vi "GoalGapToAngle.vi"(6 "x_goal":dbl, 8 "error in (no error)":errorcluster, 9 "GoalGap":dbl[](array[numeric]), 10 "Ball":refnum<class "Ball.lvclass">, 11 "object in":refnum<class "Utilities.lvclass">) -> (0 "error out":errorcluster, 1 "angle gap":dbl[](array[numeric]), 3 "object out":refnum<class "Utilities.lvclass">)   [LabVIEW 2023, in "Utilities.lvclass"]
uses:
  Utilities.lvclass
  Ball_class/Ball.lvclass
  C:/Users/lucio/Desktop/roboime/SSL_AI/Object_class/Object.lvclass
  Object_class/Object.lvclass/Object.ctl
  Object_class/Read x.vi
  Object_class/Read y.vi
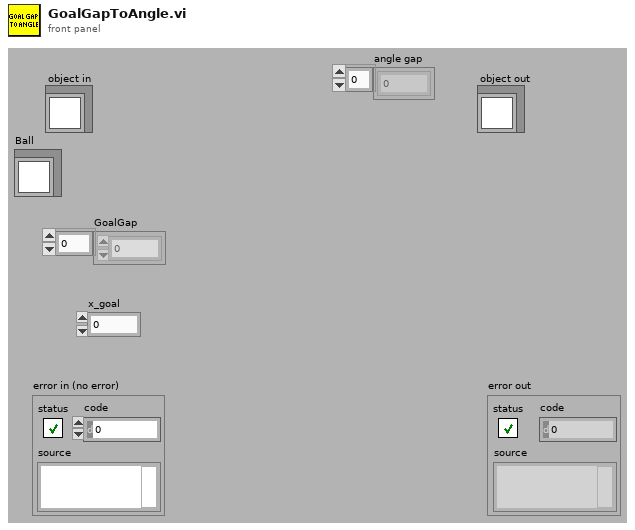
[diagram p1: front panel]
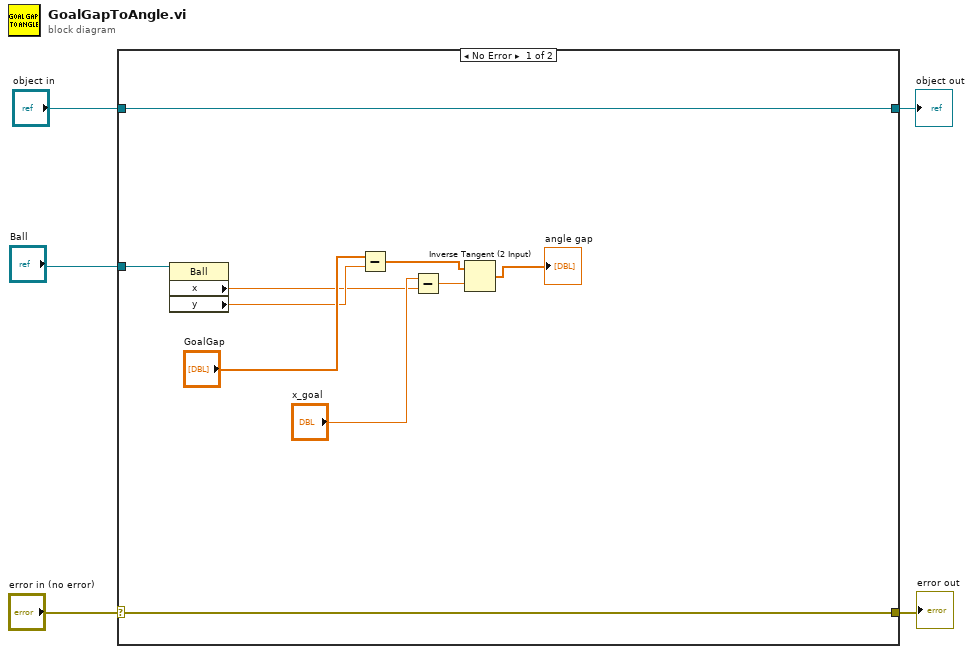
[diagram p0: block diagram]
diagram:
  n1 = case shown="No Error" "error in (no error)" {
    selector: "error in (no error)" -> [w14 w17]
    tunnel: [w14 w17] -> w4
    tunnel: [w15 w16] -> w2
    tunnel: "object in" -> [w15 w16]
    tunnel: "Ball" -> [w13 _]
    frame No Error {
      n2 = property class="Ball"(reference=w13) -> ("x"=w9:dbl, "y"=w11:dbl)  [unwired: 1 in, 2 out]
      n3 = Subtract(x="GoalGap", y=w11) -> (x-y=w7:dbl[])
      n4 = Subtract(x="x_goal", y=w9) -> (x-y=w8:dbl)
      n5 = Inverse Tangent (2 Input)(1:w8, 2:w7) -> (0:→"angle gap":dbl[])
    }
    frame Error {
    }
  }
  "error out" <- w4
  "object out" <- w2
